vi "for_v0_v11.vi"() -> ()   [LabVIEW 2009]
panel:
  in  "Start":bool
  in  "Stop":bool
  out "Gauge":dbl(knob)=9.0 scale=0.0..9.0
  out "L6":bool=TRUE
  out "L4":bool=TRUE
  out "L5":bool
  out "L7":bool=TRUE
  out "L3":bool=TRUE
  out "L2":bool=TRUE
  out "L1":bool=TRUE
  # "Stop"
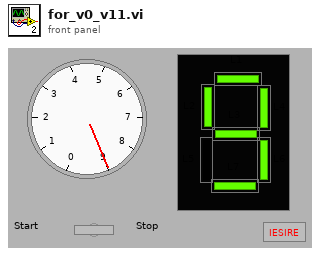
[diagram p1: front panel]
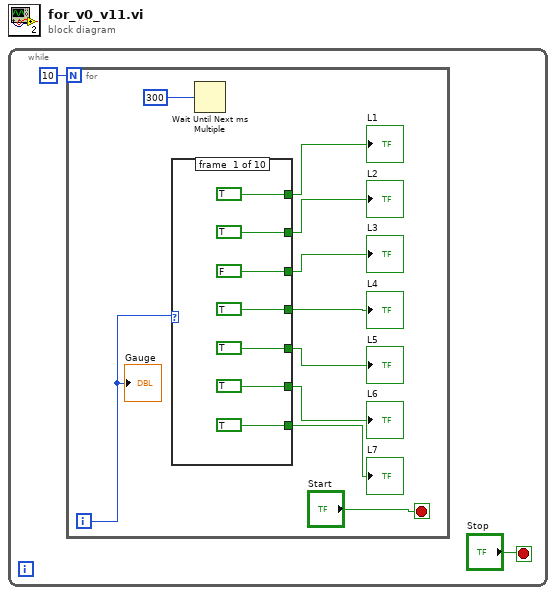
[diagram p0: block diagram]
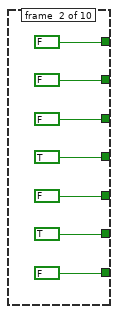
[diagram p2: hidden frame]
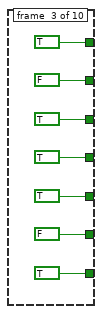
[diagram p3: hidden frame]
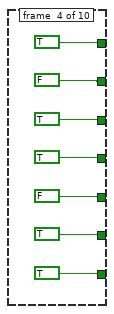
[diagram p4: hidden frame]
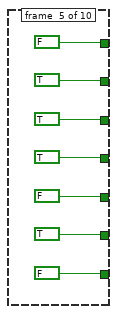
[diagram p5: hidden frame]
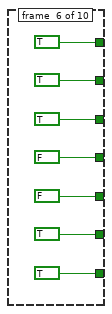
[diagram p6: hidden frame]
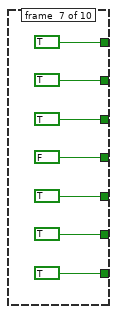
[diagram p7: hidden frame]
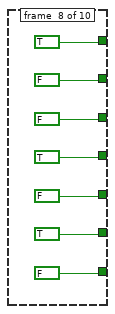
[diagram p8: hidden frame]
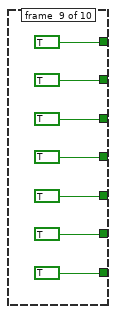
[diagram p9: hidden frame]
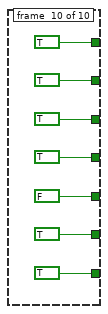
[diagram p10: hidden frame]
diagram:
  n1 = while {
    stop <- "Stop" stop-if-true
    n2 = for {
      N: 10 -> [_]
      i -> [w4]
      stop <- "Start" stop-if-true
      n3 = case shown="8" w4 {
        tunnel: [TRUE FALSE TRUE TRUE FALSE TRUE TRUE TRUE TRUE TRUE] -> w12
        tunnel: [TRUE FALSE FALSE FALSE TRUE TRUE TRUE FALSE TRUE TRUE] -> w11
        tunnel: [FALSE FALSE TRUE TRUE TRUE TRUE TRUE FALSE TRUE TRUE] -> w10
        tunnel: [TRUE TRUE TRUE TRUE TRUE FALSE FALSE TRUE TRUE TRUE] -> w9
        tunnel: [TRUE FALSE TRUE FALSE FALSE FALSE TRUE FALSE TRUE FALSE] -> w8
        tunnel: [TRUE TRUE FALSE TRUE TRUE TRUE TRUE TRUE TRUE TRUE] -> w7
        tunnel: [TRUE FALSE TRUE TRUE FALSE TRUE TRUE FALSE TRUE TRUE] -> w6
        frame #0 {
        }
        frame #1 {
        }
        frame #2 {
        }
        frame #3 {
        }
        frame #4 {
        }
        frame #5 {
        }
        frame #6 {
        }
        frame #7 {
        }
        frame #8 {
        }
        frame #9 {
        }
      }
      "L1" <- w12
      "L2" <- w11
      "L3" <- w10
      "L7" <- w6
      "L5" <- w8
      "L4" <- w9
      "L6" <- w7
      n4 = Wait Until Next ms Multiple(millisecond multiple=u32 300 ("milliseconds to wait")) -> ()  [unwired: 1 out]
      "Gauge" <- w4
    }
  }
